vi "Init Device.vi"(8 "error in (no error)":errorcluster, 11 "Virtual Microscope in":refnum<class "Virtual Microscope.lvclass">) -> (0 "error out":errorcluster, 3 "Virtual Microscope out":refnum<class "Virtual Microscope.lvclass">)   [LabVIEW 2018, in "Virtual Microscope.lvlib" / "Virtual Microscope.lvclass"]
uses:
  Virtual Microscope.lvclass
  C:/Program Files/National Instruments/LabVIEW 2018/vi.lib/ActorFramework/Actor/Actor.lvclass
  Virtual Microscope.lvclass/Virtual Microscope.ctl
  Ti2/Ti2.lvclass
  Device/Device.lvclass
  <vilib>/ActorFramework/Actor/Actor.lvclass
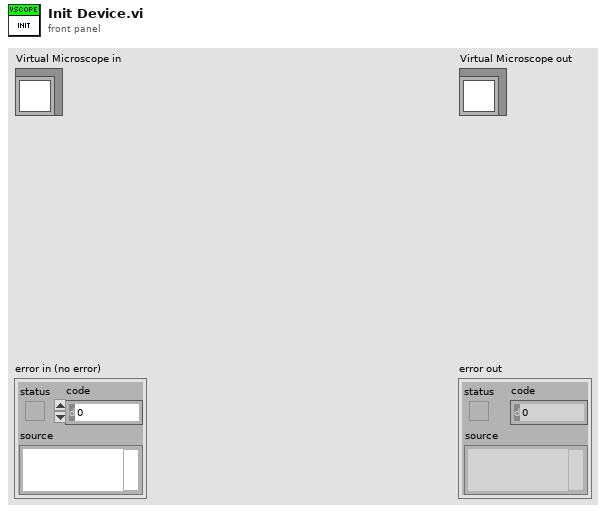
[diagram p1: front panel]
types:
  T1 = typedef "Microscope Configuration.ctl" = cluster{"Serial Port":refnum<visa-resource-name>, "Microscope Type":T2, "Detection Settings":cluster{"Name":string, "Filter Position":u16, "Optical Path":u16}[]}
  T2 = typedef "Microscope Type.ctl" = enum16{"Disable", "TE2000", "Eclipse Ti", "Ti2"}
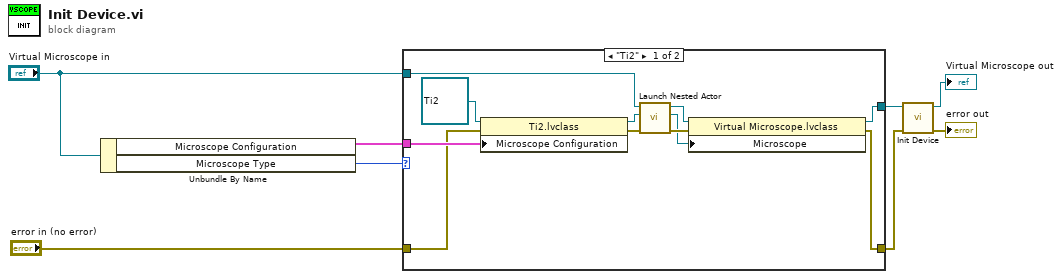
[diagram p0: block diagram]
diagram:
  n1 = Unbundle By Name("Virtual Microscope in") -> ("Microscope Configuration"=w6:T1, "Microscope Type"=w5:T2)
  n2 = case shown="\"Ti2\"" w5 {
    tunnel: "Virtual Microscope in" -> [w19 w20]
    tunnel: [w11 w20] -> w1
    tunnel: w6 -> [w17 _]
    tunnel: "error in (no error)" -> [w16 w21]
    tunnel: [w13 w21] -> w2
    frame "Ti2" {
      n3 = property class="Ti2.lvclass"(reference=refnum<class "Ti2.lvclass"> refnum ("Ti2.lvlib:Ti2.lvclass"), error in=w16, "Microscope Configuration"=w17) -> (reference out=w18:refnum<class "Ti2.lvclass">, error out=w15:errorcluster)
      n4 = call <vilib>:"Launch Nested Actor.vi"("error in (no error)"=w15, "Nested Actor"=w18, "Caller Actor in"=w19) -> ("error out"=w14:errorcluster, "Nested Actor's Enqueuer"=w10:refnum<class "Message Enqueuer.lvclass">, "Caller Actor out"=w12:refnum<class "Virtual Microscope.lvclass">)  [unwired: 6 in]
      n5 = property class="Virtual Microscope.lvclass"(reference=w12, error in=w14, "Microscope"=w10) -> (reference out=w11:refnum<class "Virtual Microscope.lvclass">, error out=w13:errorcluster)
    }
    frame "Disable", Default {
    }
  }
  n6 = call-parent "Init Device.vi"("error in (no error)"=w2, "Device in"=w1) -> ("error out"=→"error out":errorcluster, "Device out"=→"Virtual Microscope out":refnum<class "Virtual Microscope.lvclass">)  [unwired: 8 in]
